vi "ShortcutMenu.vi"(8 "error in":errorcluster, 9 "menu ref in":refnum<k9>, 11 "node in":refnum<class "NISE_CEF_serializable node.lvclass">) -> (0 "error out":errorcluster, 1 "menu ref out":refnum<k9>, 3 "node out":refnum<class "NISE_CEF_serializable node.lvclass">)   [LabVIEW 2013, in "NISE_CEF_serializable node.lvclass"]
doc: "Defines the behavior of the shortcut menu of the node."
uses:
  NISE_CEF_serializable node.lvclass
  Node/NISE_CEF_Node.lvclass
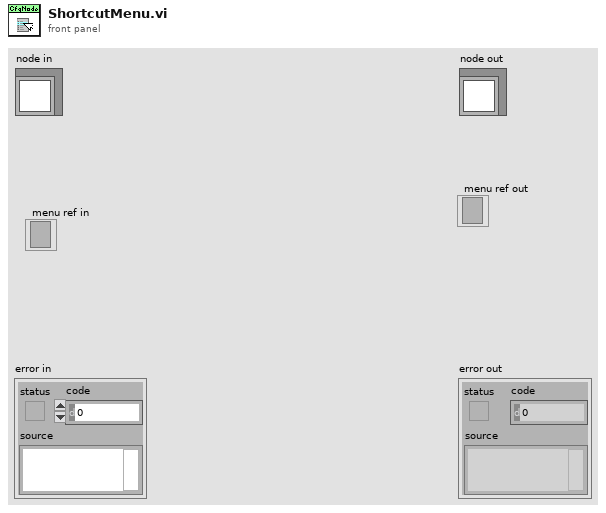
[diagram p1: front panel]
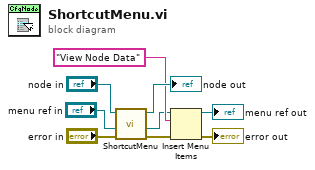
[diagram p0: block diagram]
diagram:
  n1 = call-parent "ShortcutMenu.vi"("error in"="error in", "menu ref in"="menu ref in", "node in"="node in") -> ("error out"=w1:errorcluster, "menu ref out"=w4:refnum<k9>, "node out"=→"node out":refnum<class "NISE_CEF_serializable node.lvclass">)  [unwired: 6 in]
  n2 = Insert Menu Items(6:w1, 8:"View Node Data", 9:w4) -> (0:→"error out":errorcluster, 3:→"menu ref out":refnum<k9>)  [unwired: 3 in, 1 out]
